vi "Record Assertion Result.vi"(9 "Test Result":T1, 10 "Test Method":string, 11 "Test Case Result in":T4) -> (3 "Test Case Result out":T4)   [LabVIEW 2020, in "Test Case Result.lvlib"]
uses:
  Test Case Result.lvlib
  Test Case Result.ctl
  Method Result/Method Result.ctl
  Assertion Result/Public/TypeDefs/Status.ctl
  Assertion Result/Assertion Result.ctl
  Assertion Result/Public/TypeDefs/Assertion Type.ctl
  <vilib>/Utility/miscctls.llb/LVMapReplaceAction.ctl
  Method Result/Private/Merge Status.vi
  Method Result/Private/Concatenate result strings.vi
  Method Result/Method Result.lvlib
  Assertion Result/Assertion Result.lvlib
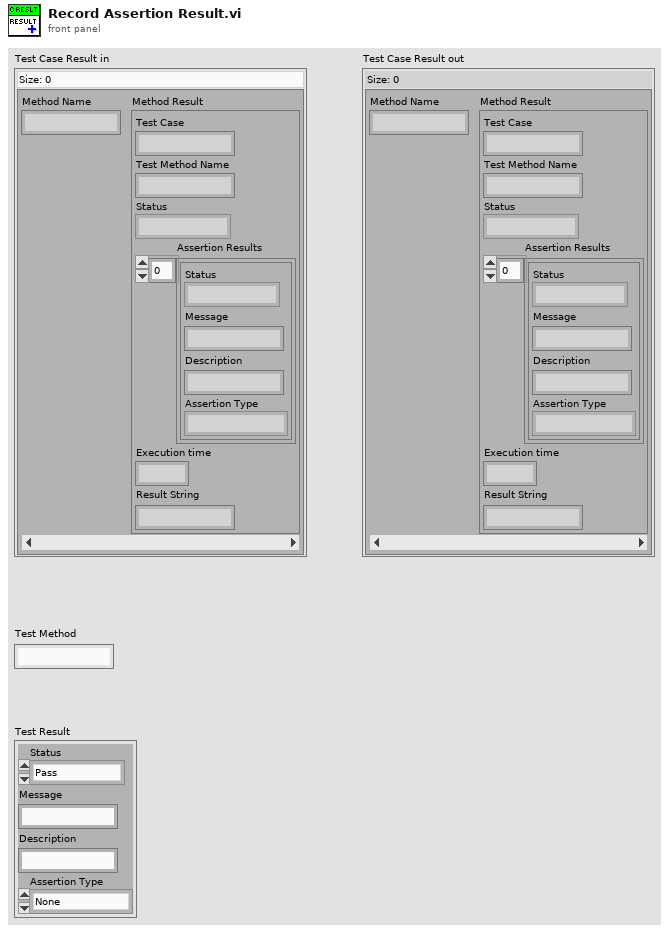
[diagram p1: front panel]
types:
  T1 = typedef "Assertion Result.lvlib/Assertion Result.ctl" = cluster{"Status":T2, "Message":string, "Description":string, "Assertion Type":T3}
  T2 = typedef "Assertion Result.lvlib/Status.ctl" = enum16{"Pass", "Fail", "Error", "Skipped", "Setup Error", "Broken", "Teardown Error"}
  T3 = typedef "Assertion Result.lvlib/Assertion Type.ctl" = enum16{"None", "Pass", "Fail", "Skip", "Pass if Equal", "Fail if Equal", "Pass if Error", "Fail if Error", "Pass if", "Fail if"}
  T4 = typedef "Test Case Result.lvlib/Test Case Result.ctl" = map{string, T5}
  T5 = typedef "Method Result.lvlib/Method Result.ctl" = cluster{"Test Case":string, "Test Method Name":string, "Status":T2, "Assertion Results":T1[], "Execution time":dbl, "Result String":string}
  T6 = typedef "LVMapReplaceAction.ctl" = enum32{"Modify Entry only if found", "Add or Modify Entry", "Delete Entry"}
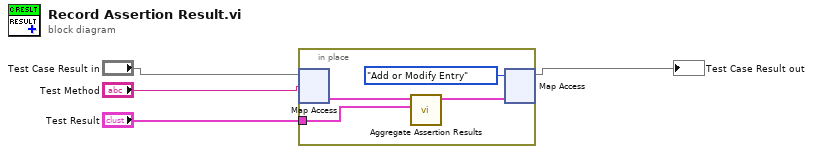
[diagram p0: block diagram]
diagram:
  n1 = in-place {
    in-place-border: "Test Result" -> [w6]
    n2 = in-place-map #1("Test Case Result in", "Test Method") -> (w8:T5)  [unwired: 1 in, 1 out]
    n3 = call "Aggregate Assertion Results.vi"("Assertion Result"=w6, "Method Result In"=w8) -> ("Method Result Out"=w7:T5)  [unwired: 9 in]
    n4 = in-place-map #1(w7, LVMapReplaceAction."Add or Modify Entry" ("action")) -> (→"Test Case Result out":T4)  [unwired: 2 out]
  }
